vi "Pockels-Ref scan cycles.vi"() -> (1 "Ref Scan Cycles":i32, 3 "Adjusted time between ref \ntriggers sent to the FPGA (ms)":dbl)   [LabVIEW 2020]
uses:
  Globals/gl_Pockels control globals.vi
panel:
  in  "Fine tuning multiplier for POI case":dbl=1.0 format="%#_13g"
  # "<-- This is the time between reference frame triggers in FPGA clock cycles"
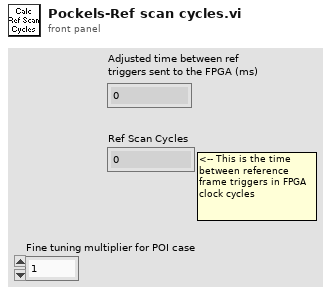
[diagram p1: front panel]
types:
  T1 = typedef "AOL_Globals.ctl" = cluster{"Imaging Protocol":T2, "Number of POI":u16, "Number of Miniscans":u16, "Number of Trials":u16, "Number of Cycles ":u64, "# Averaged Frames":u16, "Laser power (%)":u8, "Pockels (V)":dbl, "Acquisition Length (sec)":dbl, "Fill time (us)":dbl, "POI Dwell time (us)":dbl, "Miniscan Dwell time per pixel (us)":dbl, "PMT 1":dbl, "PMT 2":dbl, "Back Apperture (mA)":dbl, "Frame Size":T3, "Center Frequency":dbl, "Field of View (norm)":dbl, "DwellTime (us)":dbl, "Wavelength (nm)":dbl, "Zoom":dbl, "AOL Z":dbl, "AOL Mode":T4, "GridXY":dbl, "GridZ":dbl, "TriggerPeriod (sec)":dbl, "Number of Pixels in Miniscan":u16, "Experiment folder path":path, "X centre":dbl, "Y centre":dbl, "Angle (degrees)":dbl, "Plane Mode":T5, "Threshold":u16[], "Regenerate Chirps":bool, "Rectangle ROI length (pixels)":u16, "Rectangle ROI height (pixels)":u16, "AOD fill":u16, "StartupDelay":i32, "Samples Wait after Trigger":u16, "Slip Cycle":u32, "Add Cycle":bool, "Functional Mode":T6, "Z Start":dbl, "Z Stop":dbl, "# Planes":i32, "Total Pixels":i32, "Variable Miniscan Pixels":u16[], "Use Variable Length":bool, "Use Variable Resolution":bool, "Laser power (%) at Z Start":u8, "Laser power (%) at Z Stop":u8, "Ref Z Step":i8, "Ref Dwell Time (us)":dbl, "Field of View (um)":dbl}
  T2 = typedef "Imaging Protocols enum.ctl" = enum16{"AOL Z-Stack", "Motor Z Stack", "Functional Acquisition", "Single Plane Acquisition", "Volume Acquisition", "Live Imaging", "Live Plane Imaging", "Live Volume Imaging"}
  T3 = typedef "Frame Size.ctl" = u16
  T4 = typedef "AOL modes.ctl" = enum16{"Raster", "Structural", "Pointing", "Mini Scan", "Alignment"}
  T5 = typedef "Plane Mode.ctl" = u16
  T6 = typedef "Functional Mode.ctl" = enum16{"Point", "Line", "Patch", "Plane", "Volume"}
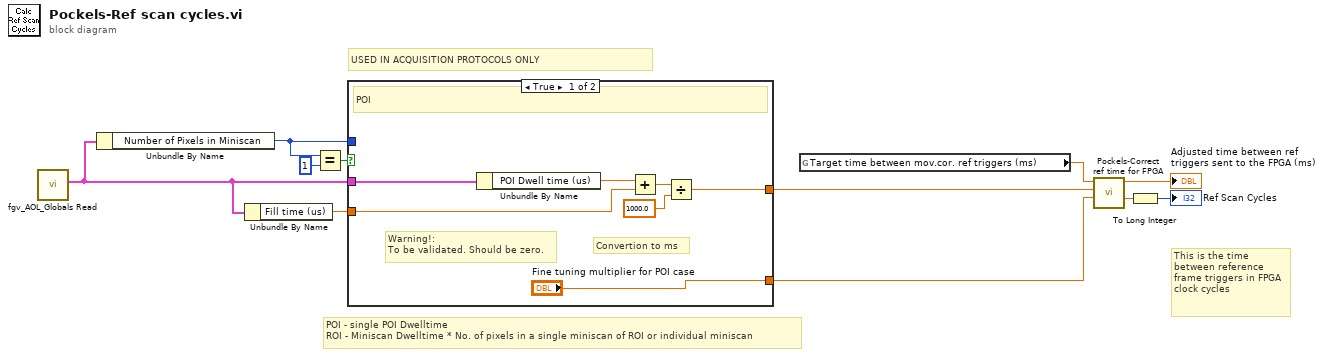
[diagram p0: block diagram]
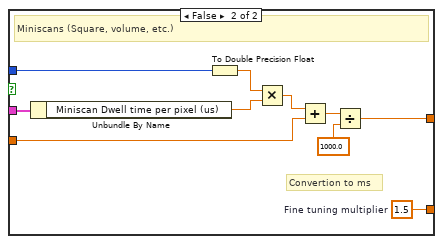
[diagram p2: hidden frame]
diagram:
  # "POI - single POI Dwelltime\nROI - Miniscan Dwelltime * No. of pixels in a single miniscan of ROI or individual miniscan"
  # "USED IN ACQUISITION PROTOCOLS ONLY"
  # "This is the time between reference frame triggers in FPGA clock cycles"
  n1 = call "fgv_AOL_Globals Read.vi"() -> ("AOL_Globals"=w4:T1)  [unwired: 9 in, 2 out]
  n2 = Unbundle By Name(w4) -> ("Number of Pixels in Miniscan"=w5:u16)
  n3 = Unbundle By Name(w4) -> ("Fill time (us)"=w3:dbl)
  n4 = Equal?(x=w5, y=u16 1) -> (x = y?=w6:bool)
  n5 = case shown="True" w6 {
    tunnel: [w18 w28] -> w9
    tunnel: w4 -> [w15 w25]
    tunnel: w5 -> [_ w23]
    tunnel: w3 -> [w13 w20]
    tunnel: ["Fine tuning multiplier for POI case" w19] -> w1
    frame True {
      # "Warning!:\nTo be validated. Should be zero."
      # "Convertion to ms"
      # "POI"
      n6 = Unbundle By Name(w15) -> ("POI Dwell time (us)"=w14:dbl)
      n7 = Add(x=w14, y=w13) -> (x+y=w17:dbl)
      n8 = Divide(x=w17, y=1000.0) -> (x/y=w18:dbl)
    }
    frame False {
      w19 = 1.5  # Fine tuning multiplier
      # "Convertion to ms"
      # "Miniscans (Square, volume, etc.)"
      n9 = Unbundle By Name(w25) -> ("Miniscan Dwell time per pixel (us)"=w24:dbl)
      n10 = To Double Precision Float(number=w23) -> (double precision float=w21:dbl)
      n11 = Multiply(x=w21, y=w24) -> (x*y=w22:dbl)
      n12 = Add(x=w22, y=w20) -> (x+y=w27:dbl)
      n13 = Divide(x=w27, y=1000.0) -> (x/y=w28:dbl)
    }
  }
  n14 = global read "gl_Pockels control globals.vi" "Target time between mov.cor. ref triggers (ms)"() -> (w2:dbl)
  n15 = call "Pockels-Correct ref time for FPGA.vi"("Fine tuning multiplier"=w1, "Time for main img line OR for a single POI (ms)"=w9, "Actual resulting time between ref triggers (ms)"=w2) -> ("Ref Scan Cycles"=w10:dbl, "Adjusted time between ref \ntriggers sent to the FPGA (ms)"=→"Adjusted time between ref \ntriggers sent to the FPGA (ms)":dbl)  [unwired: 7 in]
  n16 = To Long Integer(number=w10) -> (32bit integer=→"Ref Scan Cycles":i32)
